vi "failure_voltage.vi"() -> ()   [LabVIEW 2023]
panel:
  out "Failure Voltage (V)":dbl
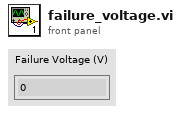
[diagram p1: front panel]
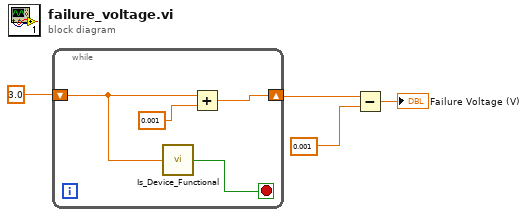
[diagram p0: block diagram]
diagram:
  n1 = while {
    shift-right: [w6] -> w2
    shift-left: 3.0 -> [w5]
    stop <- w8 stop-if-true
    n2 = call "Is_Device_Functional.vi"("Operating_Voltage(V)"=w5) -> ("Device_Functional"=w8:bool)  [unwired: 14 in]
    n3 = Add(x=w5, y=0.001) -> (x+y=w6:dbl)
  }
  n4 = Subtract(x=w2, y=0.001) -> (x-y=→"Failure Voltage (V)":dbl)
